vi "RSZVB Get Source Combiner State.vi"(8 "error in (no error)":errorcluster {"code" format="%.0x"}, 10 "Channel (1)":i32=1, 11 "VISA session":refnum<visa-resource-name>) -> (0 "error out":errorcluster {"code" format="%.0x"}, 2 "State":bool, 3 "dup VISA session":refnum<visa-resource-name>)   [LabVIEW 2011]
doc: "This VI returns the source combiner for reference channel.\n\n\nNotes:\n\n(1) This VI is available only with hardware option B11.\n\nRemote-control command(s):\nSOURce<Ch>:POWer:COMBiner?"
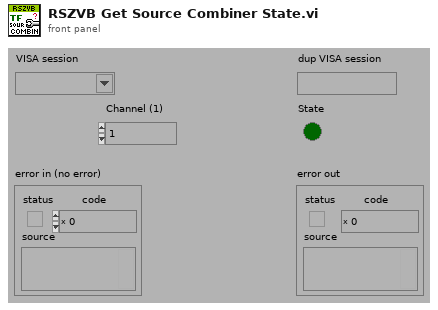
[diagram p1: front panel]
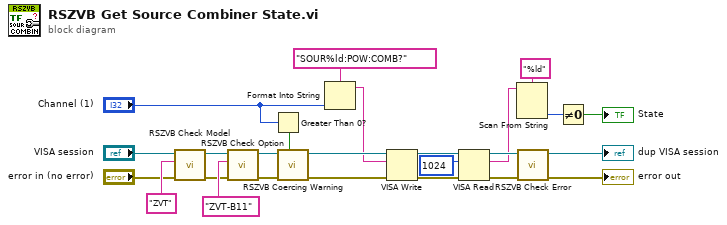
[diagram p0: block diagram]
diagram:
  n1 = call "RSZVB Check Model.vi"("error in (no error)"="error in (no error)", "Model"="ZVT" ("Options"), "VISA session"="VISA session") -> ("error out"=w17:errorcluster, "dup VISA session"=w16:refnum<visa-resource-name>)  [unwired: 7 in]
  n2 = call "RSZVB Check Option.vi"("error in (no error)"=w17, "Options"="ZVT-B11", "VISA session"=w16) -> ("error out"=w18:errorcluster, "dup VISA session"=w15:refnum<visa-resource-name>)  [unwired: 7 in]
  n3 = Greater Than 0?(x="Channel (1)") -> (x > 0?=w21:bool)
  n4 = call "RSZVB Coercing Warning.vi"("In Range?"=w21, "error in (no error)"=w18, "VISA session"=w15) -> ("error out"=w23:errorcluster, "dup VISA session"=w24:refnum<visa-resource-name>)  [unwired: 7 in]
  n5 = Format Into String(format string="SOUR%ld:POW:COMB?", "Channel (1)") -> (resulting string=w22:string)  [unwired: 2 in, 1 out]
  n6 = VISA Write(VISA resource name=w24, write buffer=w22, error in (no error)=w23) -> (VISA resource name out=w6:refnum<visa-resource-name>, error out=w7:errorcluster)  [unwired: 1 out]
  n7 = VISA Read(VISA resource name=w6, byte count=u32 1024 ("byte count (0)"), error in (no error)=w7) -> (VISA resource name out=w12:refnum<visa-resource-name>, read buffer=w10:string, error out=w11:errorcluster)  [unwired: 1 out]
  n8 = Scan From String(format string="%ld", input string=w10) -> (output 1=w9:i32)  [unwired: 3 in, 3 out]
  n9 = call "RSZVB Check Error.vi"("error in (no error)"=w11, "VISA session"=w12) -> ("error out"=→"error out":errorcluster, "dup VISA session"=→"dup VISA session":refnum<visa-resource-name>)  [unwired: 8 in]
  n10 = Not Equal To 0?(x=w9) -> (x != 0?=→"State":bool)
